vi "Sub_time_constant_start_2022.vi"(0 "time_frequency_calculations_start":dbl[](array[numeric]), 1 "time_accelerometer_acquire_start":dbl[](array[numeric]), 2 "Experimental Results IN":T1={"time_average_cycle"=0.0, "measured_frequency"=[], "date_time"="", "estimated_pin_node"=[], "time_cycle_start"=[], "measured_pin_location"=[], "estimated_frequency"=[], "acceleration_data"=[], "accelerometer_sample_rate"=0.0, "displacement_sample_rate"=0.0, "time_compare_start"=array[564 elements], "time_subsample_start"=array[564 elements], "time_FEA_start"=array[564 elements], "time_FEA_end"=array[564 elements], "time_cycle_end"=array[564 elements], "time_accelerometer_aquire_start"=array[564 elements], "time_frequency_calculations_start"=array[564 elements], "time_frequency_calculations_end"=array[564 elements], "measured_pin_location_tt"=array[564 elements], "time_ACC_data_collection_start"=0.0, "time_acceleration_data"=array[564 elements], "estimated_pin_location"=array[564 elements], "scaling_factor_Hz_per_pin_to_frequency_resolution"=1.0, "Std_Dev_equale_particles_divided_3"=TRUE, "Auto_FFT_length"=TRUE, "windowed_acc_data"=array1x564[564 elements], "FFT"=array1x564[564 elements]}, 3 "time_subsample_start":dbl[](array[numeric]), 4 "time_FEA_end":dbl[](array[numeric]), 6 "time_frequency_calculations_end":dbl[](array[numeric]), 7 "time_compare_start":dbl[](array[numeric]), 8 "measured_pin_location_tt":dbl[](array[numeric]), 9 "time_cycle_end":dbl[](array[numeric]), 11 "time_cycle_start":dbl[](array[numeric]), 13 "time_FEA_start":dbl[](array[numeric])) -> (16 "Experimental Results OUT":T1={"time_average_cycle"=0.0, "measured_frequency"=[], "date_time"="", "estimated_pin_node"=[], "time_cycle_start"=[], "measured_pin_location"=[], "estimated_frequency"=[], "acceleration_data"=[], "accelerometer_sample_rate"=0.0, "displacement_sample_rate"=0.0, "time_compare_start"=array[564 elements], "time_subsample_start"=array[564 elements], "time_FEA_start"=array[564 elements], "time_FEA_end"=array[564 elements], "time_cycle_end"=array[564 elements], "time_accelerometer_aquire_start"=array[564 elements], "time_frequency_calculations_start"=array[564 elements], "time_frequency_calculations_end"=array[564 elements], "measured_pin_location_tt"=array[564 elements], "time_ACC_data_collection_start"=0.0, "time_acceleration_data"=array[564 elements], "estimated_pin_location"=array[564 elements], "scaling_factor_Hz_per_pin_to_frequency_resolution"=1.0, "Std_Dev_equale_particles_divided_3"=TRUE, "Auto_FFT_length"=TRUE, "windowed_acc_data"=array1x564[564 elements], "FFT"=array1x564[564 elements]})   [LabVIEW 2021]
uses:
  <vilib>/Analysis/baseanly.llb/Mean (DBL).vi
  <vilib>/Analysis/NI_AALBase.lvlib
panel:
  out "mean":dbl format="%0.10f"
  out "number of iterations run":i32
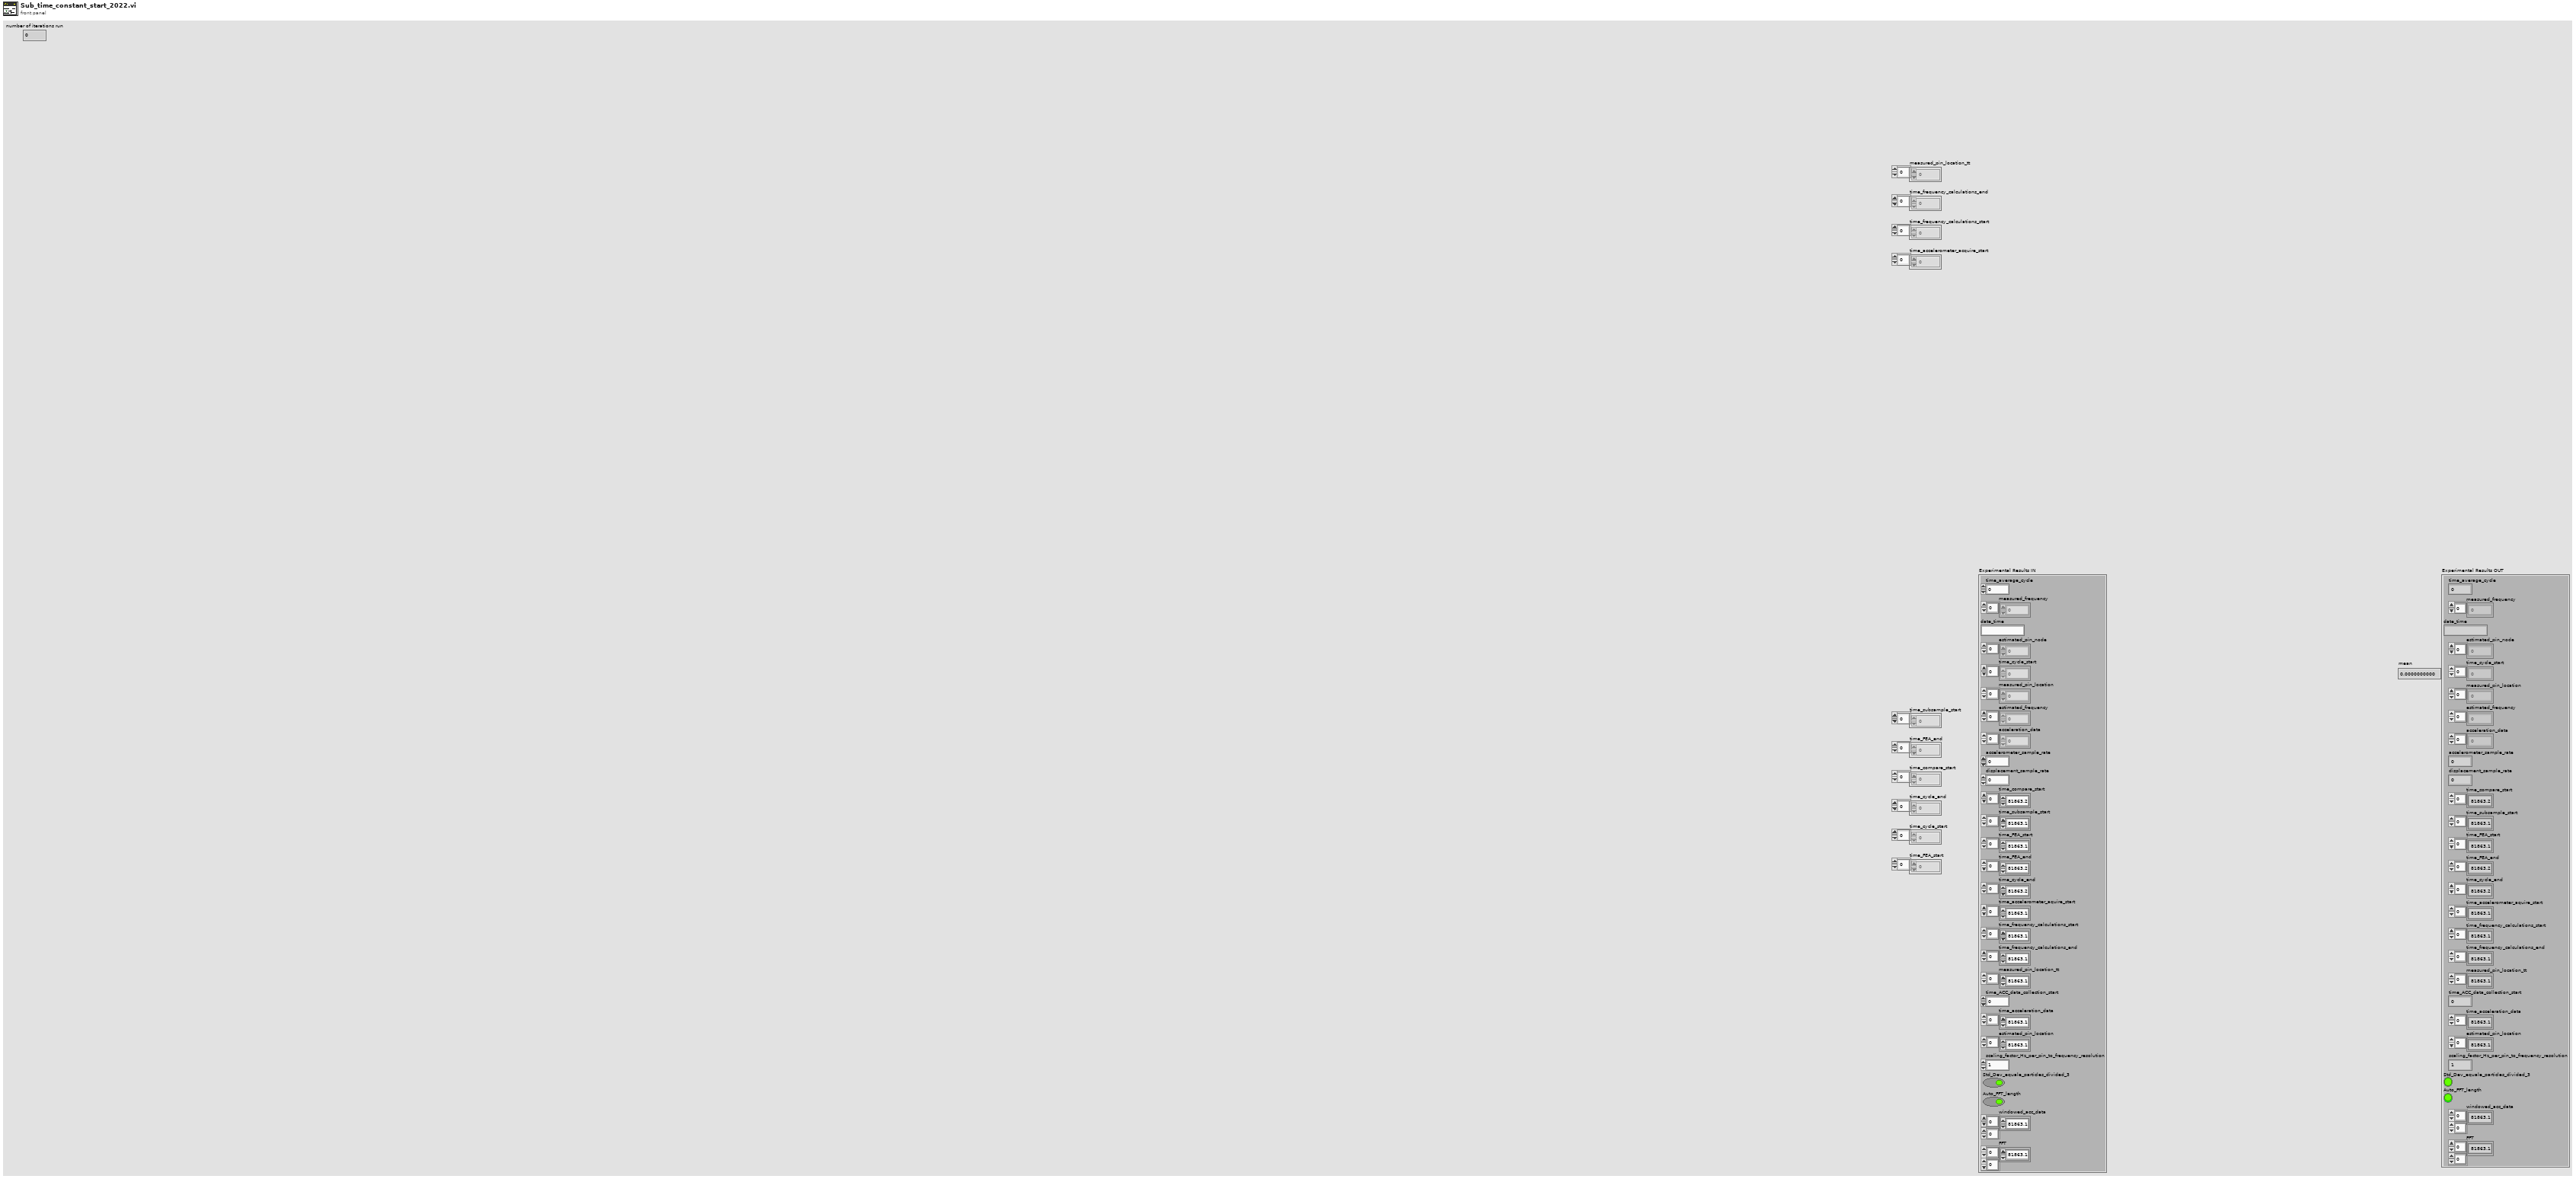
[diagram p1: front panel]
types:
  T1 = cluster{"time_average_cycle":dbl, "measured_frequency":dbl[], "date_time":string, "estimated_pin_node":i32[], "time_cycle_start":dbl[], "measured_pin_location":dbl[], "estimated_frequency":dbl[], "acceleration_data":dbl[], "accelerometer_sample_rate":dbl, "displacement_sample_rate":dbl, "time_compare_start":dbl[], "time_subsample_start":dbl[], "time_FEA_start":dbl[], "time_FEA_end":dbl[], "time_cycle_end":dbl[], "time_accelerometer_aquire_start":dbl[], "time_frequency_calculations_start":dbl[], "time_frequency_calculations_end":dbl[], "measured_pin_location_tt":dbl[], "time_ACC_data_collection_start":dbl, "time_acceleration_data":dbl[], "estimated_pin_location":dbl[], "scaling_factor_Hz_per_pin_to_frequency_resolution":dbl, "Std_Dev_equale_particles_divided_3":bool, "Auto_FFT_length":bool, "windowed_acc_data":dbl[][], "FFT":dbl[][]}
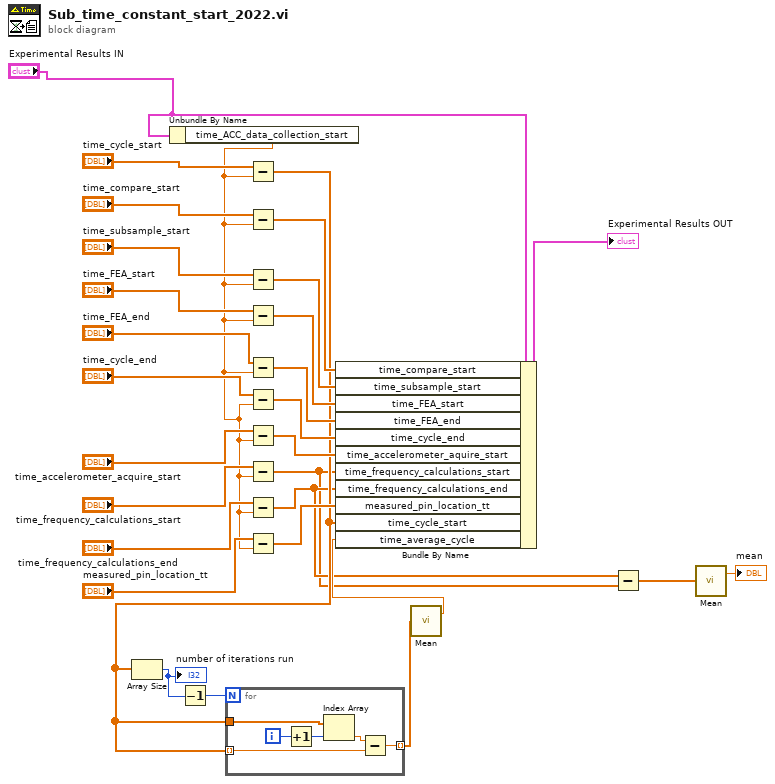
[diagram p0: block diagram]
diagram:
  n1 = Unbundle By Name("Experimental Results IN") -> ("time_ACC_data_collection_start"=w12:dbl)
  n2 = Subtract(x="time_cycle_start", y=w12) -> (x-y=w7:dbl[])
  n3 = Array Size(array=w7) -> (size(s)=w10:i32)
  "number of iterations run" <- w10
  n4 = Decrement(x=w10) -> (x-1=w11:i32)
  n5 = for {
    N: w11 -> [_]
    tunnel: w7 -> [w35] mode=indexing
    tunnel: w7 -> [w34]
    tunnel: [w30] -> w9 mode=indexing
    i -> [w33]
    n6 = Increment(x=w33) -> (x+1=w32:i32)
    n7 = Index Array(array=w34, index=w32) -> (element=w31:dbl)
    n8 = Subtract(x=w31, y=w35) -> (x-y=w30:dbl)
  }
  n9 = Subtract(x="time_compare_start", y=w12) -> (x-y=w29:dbl[])
  n10 = Subtract(x="time_subsample_start", y=w12) -> (x-y=w28:dbl[])
  n11 = Subtract(x="time_FEA_start", y=w12) -> (x-y=w27:dbl[])
  n12 = Subtract(x="time_FEA_end", y=w12) -> (x-y=w13:dbl[])
  n13 = Subtract(x="time_cycle_end", y=w12) -> (x-y=w26:dbl[])
  n14 = Subtract(x="time_accelerometer_acquire_start", y=w12) -> (x-y=w25:dbl[])
  n15 = Subtract(x="time_frequency_calculations_start", y=w12) -> (x-y=w5:dbl[])
  n16 = Subtract(x="time_frequency_calculations_end", y=w12) -> (x-y=w6:dbl[])
  n17 = Subtract(x="measured_pin_location_tt", y=w12) -> (x-y=w24:dbl[])
  n18 = call-poly <vilib>:"Mean.vi"("X"=w9) -> ("mean"=w8:dbl)  [unwired: 1 out]
  n19 = Bundle By Name(cluster="Experimental Results IN", "time_compare_start"=w29, "time_subsample_start"=w28, "time_FEA_start"=w27, "time_FEA_end"=w13, "time_cycle_end"=w26, "time_accelerometer_aquire_start"=w25, "time_frequency_calculations_start"=w5, "time_frequency_calculations_end"=w6, "measured_pin_location_tt"=w24, "time_cycle_start"=w7, "time_average_cycle"=w8) -> (→"Experimental Results OUT":T1)
  n20 = Subtract(x=w6, y=w5) -> (x-y=w4:dbl[])
  n21 = call-poly <vilib>:"Mean.vi"("X"=w4) -> ("mean"=→"mean":dbl)  [unwired: 1 out]
